vi "Game Controller Teleop.vi"(10 "Match Info":T13={"Autonomous Elapsed Seconds"=0.0, "TeleOp Elapsed Seconds"=0.0, "Disabled Elapsed Seconds"=0.0, "Visited Autonomous"=FALSE, "Visited TeleOp"=FALSE, "Visited Disabled"=FALSE, "Autonomous Settings"={"Autonomous Style"=enum."Independent", "VI Refnum"=refnum}}, 11 "Call Context":T14) -> ()   [LabVIEW 2020]
doc: "This VI is called for each TeleOp packet received from the DS where the robot is not disabled. It is often used to read from the joysticks and update I/O or to update setpoints for timed control loops. It should complete and return within 20 milliseconds or it may miss DS packets."
uses:
  <vilib>/Rock Robotics/WPI/DriverStation/WPI_DriverStationDerivedRobotMode.ctl
  <vilib>/Rock Robotics/WPI/DriverStation/WPI_DriverStationMatch Info.ctl
  Shared Code/TypeDefs/Cluster_Extend HW Outputs.ctl
  Shared Code/TypeDefs/Cluster_FX CloseLoop Values.ctl
  Shared Code/TypeDefs/Cluster_FX Limit Switchs.ctl
  Shared Code/TypeDefs/Cluster_FX Current Values.ctl
  Shared Code/TypeDefs/Cluster_FX Sensor Values.ctl
  Shared Code/TypeDefs/Cluster_FX Integrated Sensor Values.ctl
  Shared Code/TypeDefs/Cluster_Lift_HW Outputs.ctl
  Shared Code/TypeDefs/Cluster_Wrist HW Outputs.ctl
  Shared Code/TypeDefs/Cluster_Pose Positions.ctl
  Systems/MotionMaser/ENUM_Pose List.ctl
  Type Defs/Cluster_Pigeon Tilt Data.ctl
  Shared Code/TypeDefs/ENUM_Tilt State.ctl
  Systems/SwerveDrive/Cluster_CMD_ACT_Data.ctl
  Shared Code/TypeDefs/ENUM_Swerve_CMD_Mode Select.ctl
  Shared Code/TypeDefs/Cluster_CMD_Direction Data.ctl
  Shared Code/TypeDefs/Cluster_Module Velocity-Direction-Rotations.ctl
  Shared Code/TypeDefs/Level_Velocity plus-minus 1.ctl
  Shared Code/TypeDefs/Dial_Compase heading unit circle CCW positive.ctl
  Type Defs/NUM_Rotate Input.ctl
  Shared Code/TypeDefs/Cluster_X-Y.ctl
  Systems/PigeonIMU/Cluster_CMD_SEN_Data.ctl
  Teleop Support/ENUM_Button Select.ctl
  Teleop Support/ENUM_Axes Select.ctl
  Systems/Extention/Cluster_CMD_ACT_Data.ctl
  Shared Code/TypeDefs/ENUM_Extend_CMD_Mode Select.ctl
  Systems/Lift/Cluster_CMD_ACT_Data.ctl
  Shared Code/TypeDefs/ENUM_Lift_CMD_Mode Select.ctl
  Systems/Wrist/Cluster_CMD_ACT_Data.ctl
  Shared Code/TypeDefs/ENUM_Wrist_CMD_Mode Select.ctl
  Systems/Grabber/Cluster_CMD_ACT_Data.ctl
  Shared Code/TypeDefs/ENUM_Grabber_CMD_Mode Select.ctl
  Shared Code/TypeDefs/ENUM_Controller Buzz Select.ctl
  3c76d165-6d6f-4521-944b-83df467126d5.vi
  5b221245-1683-49e4-bbda-b419f5af282c.vi
  8735cd3c-726f-4517-be5d-f0f5cfaf1625.vi
  <vilib>/Rock Robotics/Network Tables/NT Write Boolean.vi
  Systems/Game Controller/Global_SEN_Data Out.vi
  Systems/PigeonIMU/Global_CMD_SEN_Data In.vi
  Systems/Grabber/Global_CMD_ACT_Data In.vi
  Systems/Wrist/Global_CMD_ACT_Data In.vi
  Systems/Extention/Global_ACT_Data Out.vi
  Systems/Lift/Global_ACT_Data Out.vi
  Systems/Wrist/Global_ACT_Data Out.vi
  Systems/Extention/Global_CMD_ACT_Data In.vi
  Systems/Grabber/Global_ACT_Data Out.vi
  Systems/Game Controller/Global_CMD_Data In.vi
  Systems/SwerveDrive/Global_CMD_ACT_Data In.vi
  Systems/Lift/Global_CMD_ACT_Data In.vi
  Systems/PigeonIMU/Global_SEN_Data Out.vi
  Systems/SwerveDrive/Global_ACT_Data Out.vi
  <vilib>/Comparison/Equal/Equal Functor/Equal Functor.lvclass
  Systems/Game Controller/GameController_SEN.lvlib
  Systems/SwerveDrive/SwerveDrive_ACT.lvlib
  Systems/PigeonIMU/PigeonIMU_SEN.lvlib
  Systems/Extention/Extend_ACT.lvlib
  Systems/Lift/Lift_ACT.lvlib
  Systems/Wrist/Wrist_ACT.lvlib
  Systems/Grabber/Grabber_ACT.lvlib
  Systems/MotionMaser/MotionMaster_SubCMD.lvlib
panel:
  out "Rotation Reduction":dbl
  in  "min rotation speed":dbl=0.4
  in  "Balance speed (ft/s)":dbl=10.0
  out "Sen_Pigeon_Tilt Data":T1
  out "Pose":T3
  out "Target  Position Out":T4
  in  "Min Translation Speed (ft/s)":dbl=2.0 format="%#_13g"
  in  "max rotation speed":dbl=0.4
  in  "shoulder speed":dbl=-0.3
  out "ACT_Wrist_HW Output":T5
  out "ACT_Lift_HW Outputs":T11
  out "ACT_Extend_HW Outputs":T12
  out "POSITION":bool
  in  "funny tilt button":bool
  in  "Drive Deadband":dbl=0.25 format="%#_13g"
  in  "Rotation Deadband":dbl=0.15 format="%#_13g"
  in  "Square Throttle?":bool
  in  "Square Joystick Inputs?":bool
  in  "Max Translation Speed (ft/s)":dbl=16.0 format="%#_13g"
  out "POV":i16
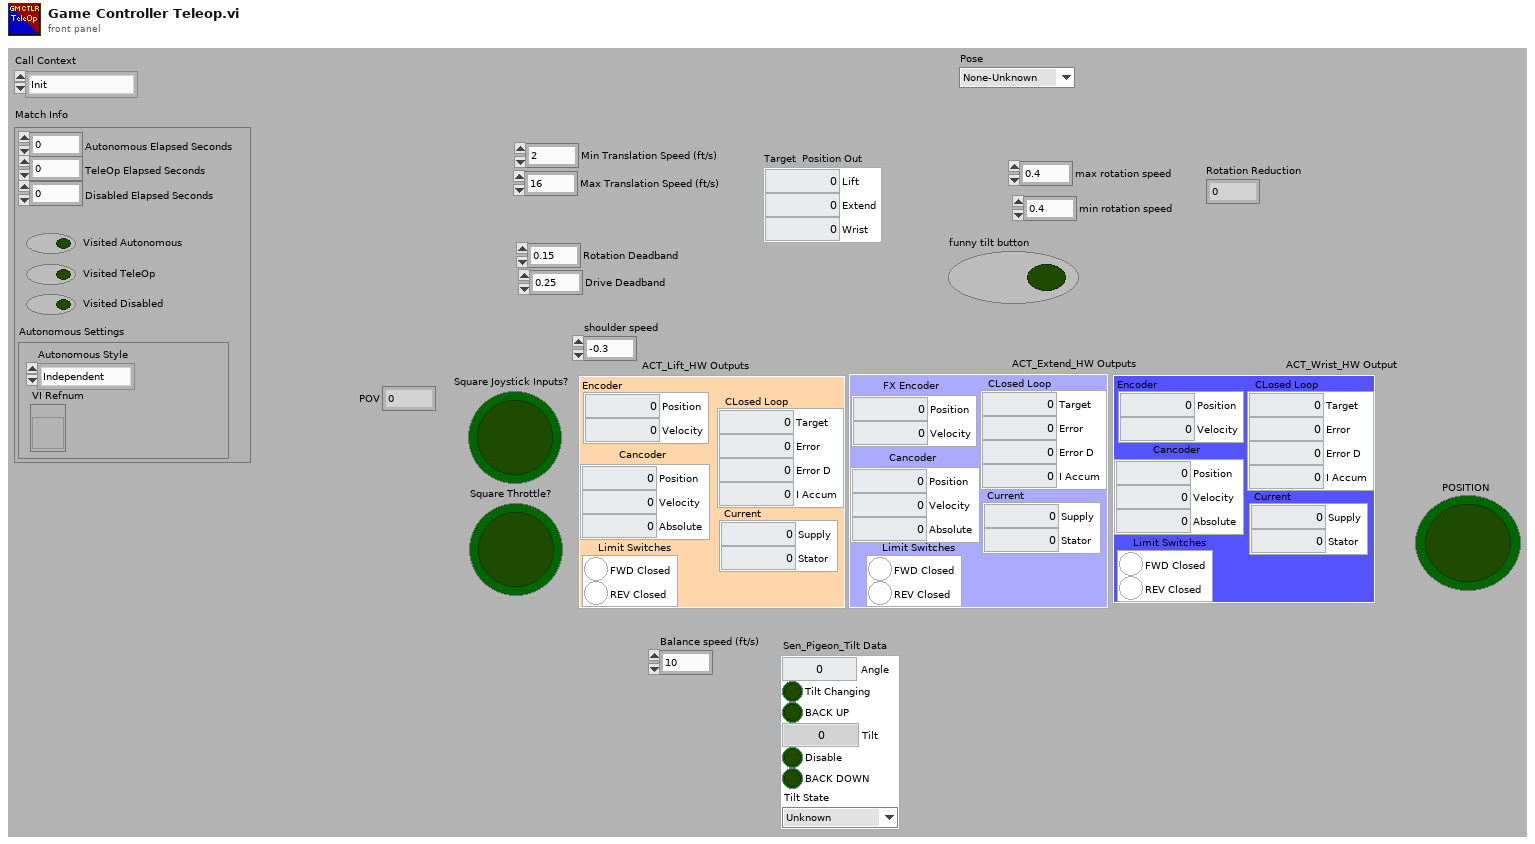
[diagram p1: front panel]
types:
  T1 = typedef "Cluster_Pigeon Tilt Data.ctl" = cluster{"Angle":dbl, "Tilt Changing":bool, "BACK UP":bool, "Tilt":dbl, "Disable":bool, "BACK DOWN":bool, "Tilt State":T2}
  T2 = typedef "ENUM_Tilt State.ctl" = enum16{"Unknown", "Level", "Angle UP from Level", "Level from Angle Up", "Angle Down from Level", "Level from Angle Down"}
  T3 = typedef "MotionMaster_SubCMD.lvlib/ENUM_Pose List.ctl" = enum16{"None-Unknown", "Intake", "Score High", "Score Mid", "Safe Position", "Home Pos"}
  T4 = typedef "Cluster_Pose Positions.ctl" = cluster{"Lift":i32, "Extend":i32, "Wrist":i32}
  T5 = typedef "Cluster_Wrist HW Outputs.ctl" = cluster{"Encoder":T6, "CLosed Loop":T7, "Limit Switches":T8, "Current":T9, "Cancoder":T10}
  T6 = typedef "Cluster_FX Sensor Values.ctl" = cluster{"Position":i32, "Velocity":i32}
  T7 = typedef "Cluster_FX CloseLoop Values.ctl" = cluster{"Target":dbl, "Error":i32, "Error D":dbl, "I Accum":dbl}
  T8 = typedef "Cluster_FX Limit Switchs.ctl" = cluster{"FWD Closed":bool, "REV Closed":bool}
  T9 = typedef "Cluster_FX Current Values.ctl" = cluster{"Supply":dbl, "Stator":dbl}
  T10 = typedef "Cluster_FX Integrated Sensor Values.ctl" = cluster{"Position":dbl, "Velocity":dbl, "Absolute":dbl}
  T11 = typedef "Cluster_Lift_HW Outputs.ctl" = cluster{"Encoder":T6, "CLosed Loop":T7, "Limit Switches":T8, "Current":T9, "Cancoder":T10}
  T12 = typedef "Cluster_Extend HW Outputs.ctl" = cluster{"CLosed Loop":T7, "Limit Switches":T8, "Current":T9, "FX Encoder":T6, "Cancoder":T10}
  T13 = typedef "WPI_DriverStationMatch Info.ctl" = cluster{"Autonomous Elapsed Seconds":dbl, "TeleOp Elapsed Seconds":dbl, "Disabled Elapsed Seconds":dbl, "Visited Autonomous":bool, "Visited TeleOp":bool, "Visited Disabled":bool, "Autonomous Settings":cluster{"Autonomous Style":enum16{"Iterative", "Independent"}, "VI Refnum":refnum<vi>}}
  T14 = typedef "WPI_DriverStationDerivedRobotMode.ctl" = enum16{"Init", "Execute", "Stop"}
  T15 = typedef "ENUM_Button Select.ctl" = enum16{"RightPad Green A", "RightPad Red B", "RightPad Blue X", "RightPad Yellow Y", "Left Bump", "Right Bump", "CenterPad Back", "CenterPad Start", "LeftStick Press", "RightStick Press"}
  T16 = typedef "ENUM_Swerve_CMD_Mode Select.ctl" = enum16{"Coast", "Manual", "Auto Trans Auto Rotate", "Manual Trans Auto Rotate", "Balance", "Stop Brake", "Lock Wheels"}
  T17 = typedef "ENUM_Extend_CMD_Mode Select.ctl" = enum16{"STOP", "Position", "Velocity", "Force Home"}
  T18 = typedef "ENUM_Axes Select.ctl" = enum16{"Left Stick Left (-1) Right (1)", "Left Stick Fwd (-1) Back(1)", "Left Trigger (0-1)", "Right Trigger (0-1)", "Right Stick Left(-1 Right (1)", "Right Stick Fwd(-1) Back (1)"}
  T19 = typedef "NUM_Rotate Input.ctl" = dbl
  T20 = typedef "Dial_Compase heading unit circle CCW positive.ctl" = dbl
  T21 = typedef "ENUM_Grabber_CMD_Mode Select.ctl" = enum16{"STOP", "Intake", "Eject"}
  T22 = typedef "Grabber_ACT.lvlib/Cluster_CMD_ACT_Data.ctl" = cluster{"Mode":T21}
  T23 = typedef "Wrist_ACT.lvlib/Cluster_CMD_ACT_Data.ctl" = cluster{"Mode":T24, "Position (counts)":i32, "Velocity (0-1)":dbl}
  T24 = typedef "ENUM_Wrist_CMD_Mode Select.ctl" = enum16{"STOP", "Position", "Speed"}
  T25 = typedef "Lift_ACT.lvlib/Cluster_CMD_ACT_Data.ctl" = cluster{"Mode":T26, "Position (counts)":i32, "Velocity (0-1)":dbl}
  T26 = typedef "ENUM_Lift_CMD_Mode Select.ctl" = enum16{"STOP", "Position", "Percent out"}
  T27 = typedef "Extend_ACT.lvlib/Cluster_CMD_ACT_Data.ctl" = cluster{"Mode":T17, "Position (counts)":i32, "Velocity (0-1)":dbl}
  T28 = typedef "PigeonIMU_SEN.lvlib/Cluster_CMD_SEN_Data.ctl" = cluster{"Reset":bool, "Disable":bool}
  T29 = typedef "Cluster_Module Velocity-Direction-Rotations.ctl" = cluster{"Velocity":T30, "Angle":T20, "Rotations Count":dbl}
  T30 = typedef "Level_Velocity plus-minus 1.ctl" = dbl
  T31 = typedef "SwerveDrive_ACT.lvlib/Cluster_CMD_ACT_Data.ctl" = cluster{"Mode":T16, "Direction":T32, "Orientation Robot(t) Field(f)":bool, "Max Translation Speed (ft/sec)":dbl, "Rotation Reduction 1-0":dbl, "Rotation Center From Robot Center":T33, "Auto Angle":T20, "Auto Target (ft)":dbl}
  T32 = typedef "Cluster_CMD_Direction Data.ctl" = cluster{"Traverse":T29, "Rotate(Yaw) CCW 1 CW -1":T19}
  T33 = typedef "Cluster_X-Y.ctl" = cluster{"X":dbl, "Y":dbl}
  T34 = typedef "Cluster_Grabber_SW Outputs.ctl" = cluster{"Enabled":bool, "Closed Loop":bool, "Stalled":bool}
  T35 = typedef "GameController_SEN.lvlib/ENUM_SEN_State.ctl" = enum16{"Startup", "Waiting BUZZ ON", "Shutdown", "Buzzing FULL Timed", "Waiting BUZZ OFF", "Buzzing Cycle Count", "Buzzing Intensity"}
  T36 = typedef "ENUM_Controller Buzz Select.ctl" = enum16{"None", "Timed Full ON", "Set Intensity", ".5 Sec Cycle Count"}
  T37 = typedef "Cluster_Config_Balance Data.ctl" = cluster{"BalancePID Ver":u64, "PID":T38}
  T38 = typedef "Cluster_PID Config.ctl" = cluster{"Gains":T39, "Error Allowed":T40, "I Zone":T40, "Max Out":T41, "Max I Accu":T40, "CL Ramp Rate (S)":dbl}
  T39 = typedef "Cluster_PID Gains.ctl" = cluster{"P":dbl, "I":dbl, "D":dbl, "F":dbl}
  T40 = typedef "Cluster_High-Low.ctl" = cluster{"High":dbl, "Low":dbl}
  T41 = typedef "Cluster_FWD  REV Values.ctl" = cluster{"FWD":dbl, "REV":dbl}
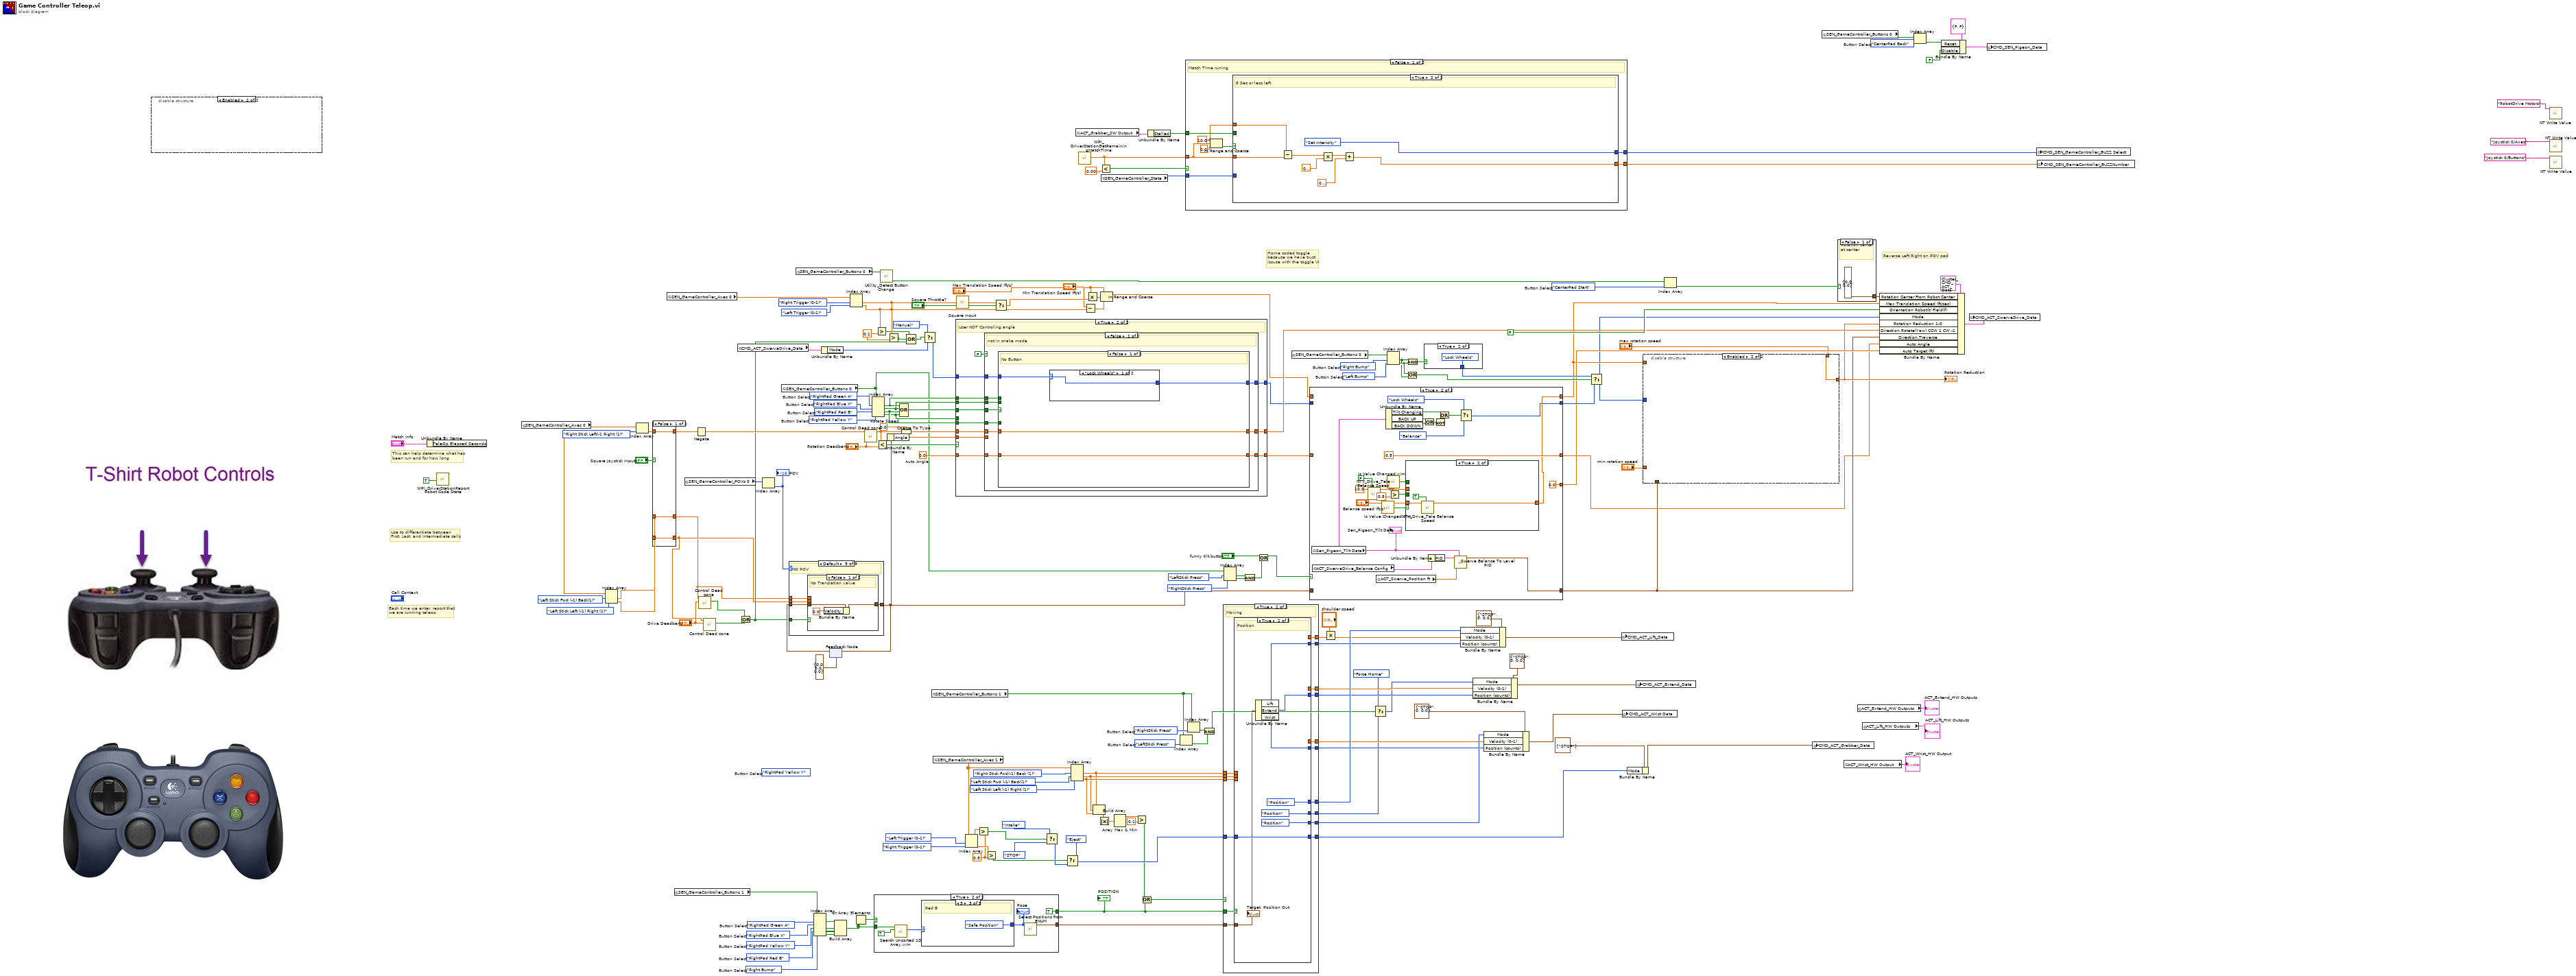
[diagram p0: block diagram]
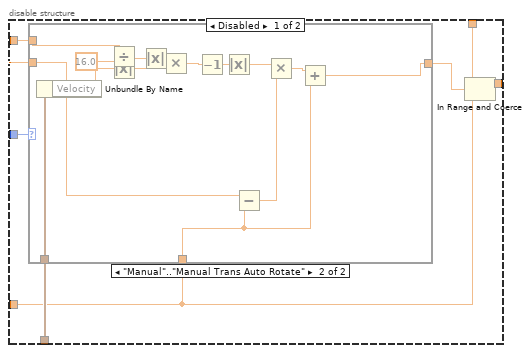
[diagram p2: hidden frame]
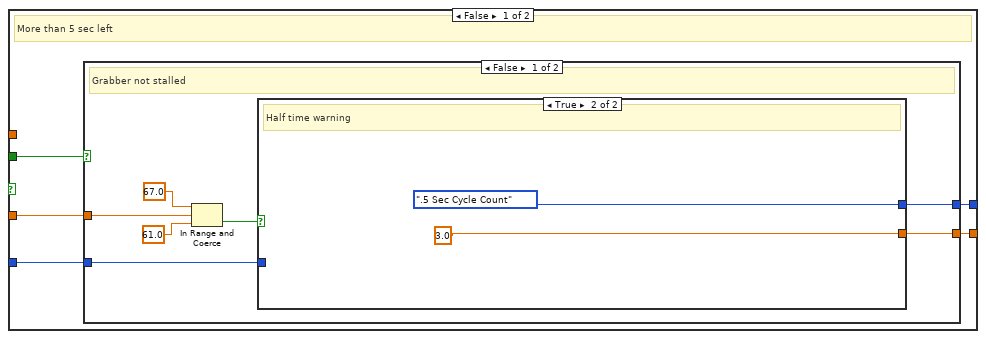
[diagram p4: hidden frame]
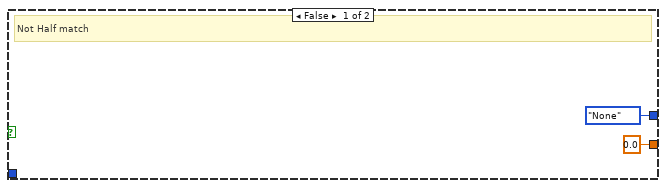
[diagram p5: hidden frame]
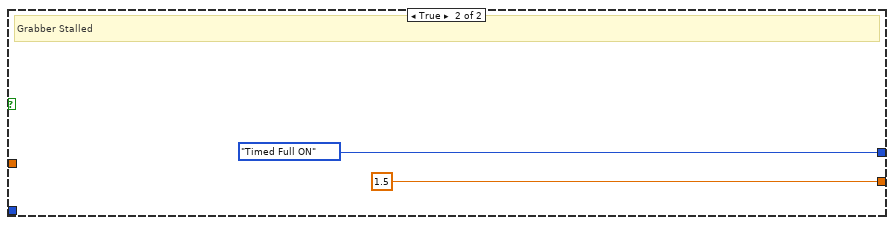
[diagram p6: hidden frame]
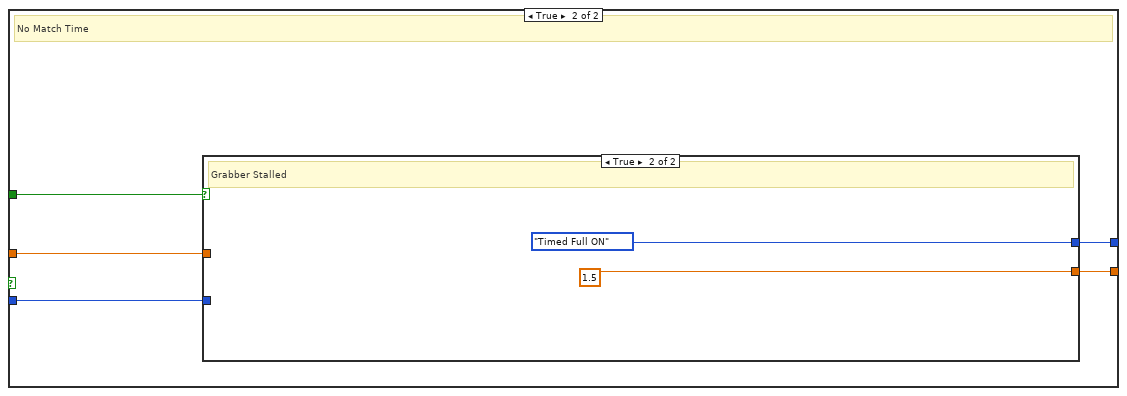
[diagram p7: hidden frame]
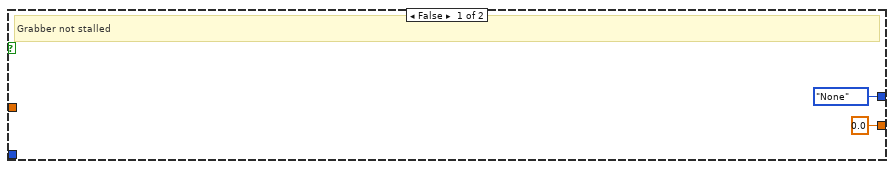
[diagram p8: hidden frame]
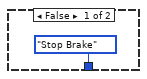
[diagram p9: hidden frame]
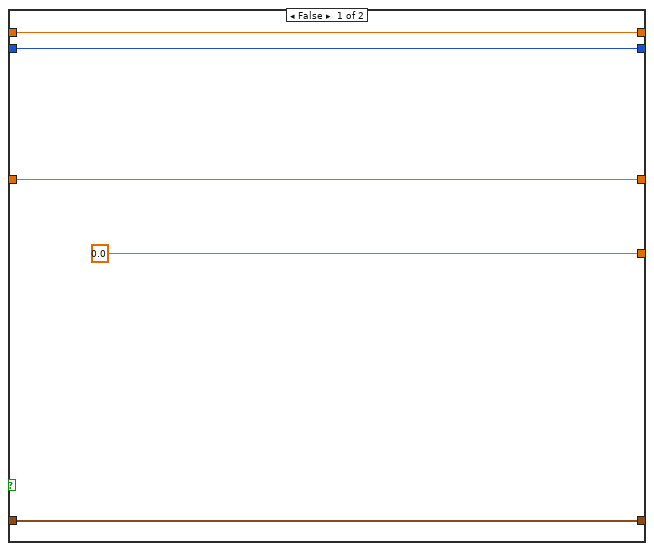
[diagram p10: hidden frame]
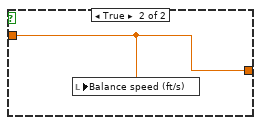
[diagram p13: hidden frame]
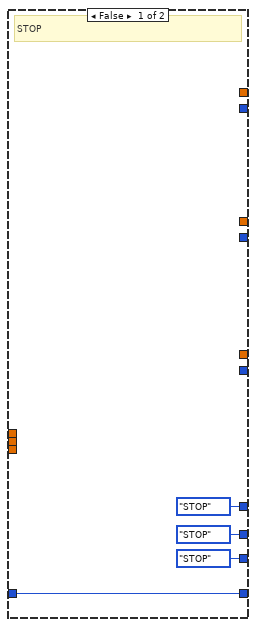
[diagram p14: hidden frame]
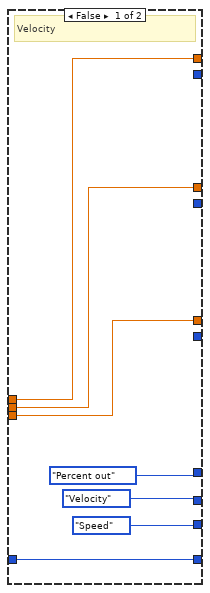
[diagram p15: hidden frame]
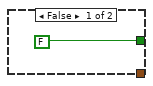
[diagram p16: hidden frame]
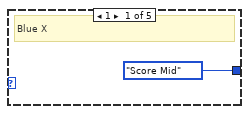
[diagram p17: hidden frame]
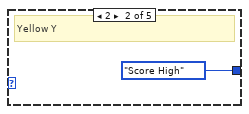
[diagram p18: hidden frame]
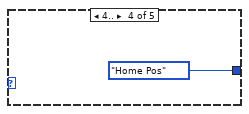
[diagram p19: hidden frame]
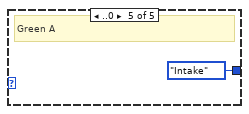
[diagram p20: hidden frame]
diagram:
  w24 = 0.1 ("y")
  w44 = ENUM_Button_Select."Left Bump"  # Button Select
  w53 = ENUM_Button_Select."LeftStick Press"  # Button Select
  w78 = T19 0.0  # Rotate Speed
  w81 = T20 0.0  # Auto Angle
  w84 = ENUM_Button_Select."Right Bump"  # Button Select
  w101 = ENUM_Button_Select."RightPad Red B"  # Button Select
  w102 = ENUM_Button_Select."RightPad Yellow Y"  # Button Select
  w103 = ENUM_Button_Select."RightPad Blue X"  # Button Select
  w104 = ENUM_Button_Select."RightPad Green A"  # Button Select
  (unwired) ENUM_Button_Select."RightPad Yellow Y"  # Button Select
  w111 = 0.9 ("y")
  w147 = ENUM_Button_Select."RightStick Press"  # Button Select
  w157 = ENUM_Button_Select."RightPad Yellow Y"  # Button Select
  w158 = ENUM_Button_Select."RightPad Red B"  # Button Select
  w159 = ENUM_Button_Select."RightPad Blue X"  # Button Select
  w167 = ENUM_Button_Select."CenterPad Start"  # Button Select
  w168 = ENUM_Button_Select."Right Bump"  # Button Select
  w172 = ENUM_Button_Select."CenterPad Back"  # Button Select
  w170 = ENUM_Button_Select."RightPad Green A"  # Button Select
  # "Home coded toggle\nbecause we have trust\nissuse with the toggle VI"
  # "Reverse Left Right on POV pad"
  # "Each time we enter, report that\nwe are running teleop"
  # "Use to differentiate between\nFirst, Last, and Intermediate calls"
  # "This can help determine what has\nbeen run and for how long"
  n1 = disable-structure shown="Enabled" {
    frame Disabled {
      n2 = global read "Global_SEN_Data Out.vi" "SEN_GameController_Axes 1"() -> (w186:dbl[])
      n3 = global read "Global_SEN_Data Out.vi" "SEN_GameController_POVs 1"() -> (w185:i16[])
      n4 = global read "Global_SEN_Data Out.vi" "SEN_GameController_Buttons 1"() -> ()  [unwired: 1 out]
      n5 = Index Array(array=w185) -> ()  [unwired: 1 in, 1 out]
      n6 = Index Array(array=w186) -> ()  [unwired: 1 in, 1 out]
    }
    frame Enabled {
    }
  }
  n7 = Unbundle By Name("Match Info") -> ()  [unwired: 1 out]
  n8 = call <vilib>:"WPI_DriverStationReport Robot Code State.vi"("TeleOp"=TRUE ("Autonomous")) -> ()  [unwired: 10 in, 1 out]
  n9 = global read "Global_SEN_Data Out.vi" "SEN_GameController_Axes 0"() -> (w140:dbl[])
  n10 = Index Array(array=w140, index #1=ENUM_Axes_Select."Left Stick Fwd (-1) Back(1)" ("Axes Select"), index #2=ENUM_Axes_Select."Left Stick Left (-1) Right (1)" ("Axes Select")) -> (element #1=w163:dbl, element #2=w136:dbl)
  n11 = Index Array(array=w140, index=ENUM_Axes_Select."Right Stick Left(-1 Right (1)" ("Axes Select")) -> (element=w138:dbl)
  n12 = case shown="False" "Square Joystick Inputs?" {
    tunnel: [w187 w190] -> w164
    tunnel: [w188 w191] -> w2
    tunnel: [w189 w192] -> w1
    tunnel: w163 -> [w189 w195]
    tunnel: w138 -> [w187 w193]
    tunnel: w136 -> [w188 w194]
    frame False {
    }
    frame True {
      n13 = call "Square Input.vi"("Input"=w193) -> ("Output Squared"=w190:dbl)
      n14 = call "Square Input.vi"("Input"=w195) -> ("Output Squared"=w192:dbl)
      n15 = call "Square Input.vi"("Input"=w194) -> ("Output Squared"=w191:dbl)
    }
  }
  n16 = global read "Global_SEN_Data Out.vi" "SEN_GameController_Axes 0"() -> (w143:dbl[])
  n17 = global read "Global_SEN_Data Out.vi" "SEN_GameController_Buttons 1"() -> (w86:bool[])
  n18 = global read "Global_SEN_Data Out.vi" "SEN_GameController_POVs 0"() -> (w179:i16[])
  n19 = Negate(x=w164) -> (-x=w75:dbl)
  n20 = call "Control Dead zone.vi"("dead zone"="Drive Deadband", "control Value"=w1) -> ("Active"=w71:bool)  [unwired: 8 in, 1 out]
  n21 = call "Control Dead zone.vi"("dead zone"="Drive Deadband", "control Value"=w2) -> ("Active"=w72:bool)  [unwired: 8 in, 1 out]
  n22 = global read "Global_CMD_ACT_Data In.vi" "CMD_ACT_SwerveDrive_Data"() -> (w29:T31)
  n23 = Or(x=w71, y=w72) -> (x .or. y?=w19:bool)
  n24 = Index Array(array=w179) -> (element=w146:i16)  [unwired: 1 in]
  "POV" <- w146
  n25 = global read "Global_SEN_Data Out.vi" "SEN_GameController_Buttons 0"() -> (w18:bool[])
  n26 = global read "Global_SEN_Data Out.vi" "SEN_GameController_Buttons 0"() -> (w55:bool[])
  n27 = Index Array(array=w86, index #1=w104, index #2=w103, index #3=w102, index #4=w101, index #5=w84) -> (element #1=w100:bool, element #2=w99:bool, element #3=w98:bool, element #4=w97:bool, element #5=w83:bool)
  n28 = Unbundle By Name(w29) -> ("Mode"=w22:T16)
  n29 = feedback #1(T29 {"Velocity"=0.0, "Angle"=0.0, "Rotations Count"=0.0} ("Polar Out")) -> (w74:T29)
  n30 = case shown="Default" w146 {
    tunnel: w1 -> [_ _ _ _ _ _ _ _ w232]
    tunnel: w2 -> [_ _ _ _ _ _ _ _ w231]
    tunnel: w74 -> [w199 w203 w207 w211 w215 w219 w223 w227 w230]
    tunnel: [w196 w200 w204 w208 w212 w216 w220 w224 w229] -> w11
    tunnel: w19 -> [_ _ _ _ _ _ _ _ w228]
    frame 0 {
      # "POV Forward"
      n31 = Bundle By Name(cluster=w199, "Velocity"=T30 1.0, "Angle"=T20 0.0) -> (w196:T29)
    }
    frame 45 {
      # "POV Forward Right"
      n32 = Bundle By Name(cluster=w203, "Velocity"=T30 1.0, "Angle"=T20 0.875) -> (w200:T29)
    }
    frame 90 {
      # "POV Right"
      n33 = Bundle By Name(cluster=w207, "Velocity"=T30 1.0, "Angle"=T20 0.75) -> (w204:T29)
    }
    frame 135 {
      # "POV Back Right"
      n34 = Bundle By Name(cluster=w211, "Velocity"=T30 1.0, "Angle"=T20 0.625) -> (w208:T29)
    }
    frame 180 {
      # "POV Back"
      n35 = Bundle By Name(cluster=w215, "Velocity"=T30 1.0, "Angle"=T20 0.5) -> (w212:T29)
    }
    frame 225 {
      # "POV Back Left"
      n36 = Bundle By Name(cluster=w219, "Velocity"=T30 1.0, "Angle"=T20 0.375) -> (w216:T29)
    }
    frame 270 {
      # "POV Left"
      n37 = Bundle By Name(cluster=w223, "Velocity"=T30 1.0, "Angle"=T20 0.25) -> (w220:T29)
    }
    frame 315 {
      # "POV Forward Left"
      n38 = Bundle By Name(cluster=w227, "Velocity"=T30 1.0, "Angle"=T20 0.125) -> (w224:T29)
    }
    frame Default {
      # "NO POV"
      n39 = case shown="False" w228 {
        tunnel: w232 -> [_ w242]
        tunnel: w231 -> [_ w241]
        tunnel: w230 -> [w234 _]
        tunnel: [w235 w238] -> w229
        frame False {
          # "No Translation value"
          n40 = Bundle By Name(cluster=w234, "Velocity"=T30 0.0) -> (w235:T29)
        }
        frame True {
          # "Tranlation Value above threshold"
          n41 = Negate(x=w241) -> (-x=w237:dbl)
          n42 = Negate(x=w242) -> (-x=w236:dbl)
          n43 = Bundle By Name(cluster=T33 {"X"=0.0, "Y"=0.0} ("XY Velocities"), "X"=w236, "Y"=w237) -> (w240:T33)
          n44 = call "Convert XY To Polar Velocities.vi"("XY Velocities"=w240) -> ("Polar Out"=w238:T29)  [unwired: 10 in]
        }
      }
    }
  }
  n45 = feedback-in #1(w11) -> ()
  n46 = Build Array(w100, w99, w98, w97, w83) -> (w95:bool[])
  n47 = Index Array(array=w143, index #1=ENUM_Axes_Select."Right Trigger (0-1)" ("Axes Select"), index #2=ENUM_Axes_Select."Left Trigger (0-1)" ("Axes Select")) -> (element #1=w27:dbl, element #2=w28:dbl)
  n48 = Or Array Elements(Boolean array=w95) -> (logical OR=w96:bool)
  n49 = call "Control Dead zone.vi"("dead zone"="Rotation Deadband", "control Value"=w75) -> ("output Value"=w80:dbl)  [unwired: 8 in, 1 out]
  n50 = Index Array(array=w18, index #1=w170, index #2=w159, index #3=w158, index #4=w157) -> (element #1=w155:bool, element #2=w152:bool, element #3=w154:bool, element #4=w153:bool)
  n51 = case shown="True" w96 {
    tunnel: [_ w245] -> w105
    tunnel: w95 -> [_ w249]
    tunnel: [FALSE TRUE] -> w61
    frame False {
    }
    frame True {
      n52 = call "Search Unsorted 1D Array.vim"("element"=TRUE, "unsorted 1D array"=w249) -> ("index of element"=w247:i32)  [unwired: 9 in]
      n53 = case shown="3" w247 {
        tunnel: [ENUM_Pose_List."Score Mid" ("Pose") ENUM_Pose_List."Score High" ("Pose") ENUM_Pose_List."Safe Position" ("Pose") ENUM_Pose_List."Home Pos" ("Pose") ENUM_Pose_List."Intake" ("Pose")] -> w244
        frame 1 {
          # "Blue X"
        }
        frame 2 {
          # "Yellow Y"
        }
        frame 3 {
          # "Red B"
        }
        frame 4.. {
        }
        frame ..0 {
          # "Green A"
        }
      }
      "Pose" <- w244
      n54 = call "Select Positions from ENUM.vi"("Pose"=w244) -> ("Selectet  Position Out"=w245:T4)  [unwired: 10 in]
    }
  }
  "POSITION" <- w61
  n55 = Greater?(x=w28, y=w24) -> (0:w25:bool)
  n56 = Less?(x=w80, y="Rotation Deadband") -> (x < y?=w150:bool)
  n57 = call "Utility_Detect Button Change.vi"("HW_Joystick_Buttons"=w55) -> ("Toggle On Rising Out"=w54:bool[])  [unwired: 6 in, 4 out]
  n58 = Greater?(x=w27, y=w24) -> (0:w26:bool)
  n59 = Unbundle By Name(w11) -> ("Angle"=w145:T20)
  n60 = Compound Arithmetic op=OR(w155, w152, w154, w153) -> (w156:bool)
  n61 = Coerce To Type(0:w80, 1:w78) -> (2:w79:T19)
  n62 = Compound Arithmetic op=OR(w25, w26, w19) -> (w23:bool)
  n63 = Select(t=ENUM_Swerve_CMD_Mode_Select."Manual", s=w23, f=w22) -> (s? t:f=w21:T16)
  n64 = global read "Global_SEN_Data Out.vi" "SEN_GameController_Buttons 1"() -> (w52:bool[])
  n65 = global read "Global_SEN_Data Out.vi" "SEN_GameController_Axes 1"() -> (w116:dbl[])
  n66 = case shown="True" w150 {
    tunnel: w79 -> [w255 w269]
    tunnel: w156 -> [_ w268]
    tunnel: w155 -> [_ w267]
    tunnel: w154 -> [_ w266]
    tunnel: w153 -> [_ _]
    tunnel: w152 -> [_ w265]
    tunnel: [w255 w264] -> w82
    tunnel: w145 -> [_ w263]
    tunnel: [ENUM_Swerve_CMD_Mode_Select."Manual" ("Mode") w260] -> w77
    tunnel: w81 -> [w256 w262]
    tunnel: [w256 w261] -> w76
    tunnel: w21 -> [_ w258]
    frame False {
      # "User Controling Angle"
    }
    frame True {
      # "User NOT Controling angle"
      n67 = case shown="False" FALSE {
        tunnel: w269 -> [w271 w303]
        tunnel: w268 -> [w277 w302]
        tunnel: w267 -> [w276 w301]
        tunnel: w266 -> [w275 w300]
        tunnel: w265 -> [w274 w299]
        tunnel: [w271 w298] -> w264
        tunnel: w263 -> [w273 _]
        tunnel: w262 -> [_ w297]
        tunnel: [w272 w296] -> w261
        tunnel: [ENUM_Swerve_CMD_Mode_Select."Manual Trans Auto Rotate" ("Mode") w295] -> w260
        tunnel: w258 -> [_ w294]
        frame True {
          # "in snake mode"
          n68 = case shown="True" w277 {
            tunnel: w276 -> [_ w284]
            tunnel: w275 -> [_ w283]
            tunnel: w274 -> [_ w282]
            tunnel: [w278 w280] -> w272
            tunnel: w273 -> [w278 w279]
            frame False {
              # "No Button"
            }
            frame True {
              # "a,b,x,y Button Pressed"
              n69 = case shown="True" w284 {
                tunnel: w283 -> [w287 _]
                tunnel: [w286 w293] -> w281
                tunnel: w282 -> [w285 _]
                frame False {
                  n70 = case shown="True" w285 {
                    tunnel: w287 -> [w289 _]
                    tunnel: [w288 w292] -> w286
                    frame False {
                      n71 = case shown="False" w289 {
                        tunnel: [w290 w291] -> w288
                        frame False {
                          w290 = T20 0.0  # Auto Angle
                          # "Y"
                        }
                        frame True {
                          w291 = T20 0.25  # Auto Angle
                          # "B"
                        }
                      }
                    }
                    frame True {
                      w292 = T20 0.75  # Auto Angle
                      # "X"
                    }
                  }
                }
                frame True {
                  w293 = T20 0.5  # Auto Angle
                  # "A"
                }
              }
              n72 = Subtract(x=w279, y=w281) -> (x-y=w280:T20)
            }
          }
        }
        frame False {
          # "not in snake mode"
          n73 = case shown="False" w302 {
            tunnel: w303 -> [w307 w311]
            tunnel: w301 -> [_ w316]
            tunnel: w300 -> [_ w315]
            tunnel: w299 -> [_ w314]
            tunnel: [w307 w311] -> w298
            tunnel: w297 -> [w306 w312]
            tunnel: [w306 w313] -> w296
            tunnel: [w305 ENUM_Swerve_CMD_Mode_Select."Manual Trans Auto Rotate" ("Mode")] -> w295
            tunnel: w294 -> [w304 _]
            frame False {
              # "No Button"
              n74 = case shown="\"Lock Wheels\"" w304 {
                selector: w304 -> [w308 _]
                tunnel: [w308 ENUM_Swerve_CMD_Mode_Select."Manual" ("Mode")] -> w305
                frame "Lock Wheels" {
                }
                frame Default {
                }
              }
            }
            frame True {
              # "a,b,x,y Button Pressed"
              n75 = case shown="True" w316 {
                tunnel: w315 -> [w320 _]
                tunnel: [w319 w327] -> w313
                tunnel: w314 -> [w318 _]
                tunnel: w312 -> [w317 _]
                frame False {
                  n76 = case shown="True" w318 {
                    tunnel: w320 -> [w323 _]
                    tunnel: [w322 w326] -> w319
                    tunnel: w317 -> [w321 _]
                    frame False {
                      n77 = case shown="True" w323 {
                        tunnel: [w324 w325] -> w322
                        tunnel: w321 -> [w324 _]
                        frame False {
                          # "Y"
                        }
                        frame True {
                          w325 = T20 0.75  # Auto Angle
                          # "B"
                        }
                      }
                    }
                    frame True {
                      w326 = T20 0.25  # Auto Angle
                      # "X"
                    }
                  }
                }
                frame True {
                  w327 = T20 0.5  # Auto Angle
                  # "A"
                }
              }
            }
          }
        }
      }
    }
  }
  n78 = call "Square Input.vi"("Input"=w27) -> ("Output Squared"=w151:dbl)
  n79 = Index Array(array=w116, index #1=ENUM_Axes_Select."Left Trigger (0-1)" ("Axes Select"), index #2=ENUM_Axes_Select."Right Trigger (0-1)" ("Axes Select")) -> (element #1=w113:dbl, element #2=w112:dbl)
  n80 = Greater?(x=w113, y=w111) -> (0:w110:bool)
  n81 = Greater?(x=w112, y=w111) -> (0:w109:bool)
  n82 = Select(t=w151, s="Square Throttle?", f=w27) -> (s? t:f=w160:dbl)
  n83 = Select(t=ENUM_Grabber_CMD_Mode_Select."Intake" ("Mode"), s=w110, f=ENUM_Grabber_CMD_Mode_Select."STOP" ("Mode")) -> (s? t:f=w117:T21)
  n84 = Select(t=ENUM_Grabber_CMD_Mode_Select."Eject" ("Mode"), s=w109, f=w117) -> (s? t:f=w94:T21)
  n85 = Index Array(array=w116, index #1=ENUM_Axes_Select."Right Stick Fwd(-1) Back (1)" ("Axes Select"), index #2=ENUM_Axes_Select."Left Stick Fwd (-1) Back(1)" ("Axes Select"), index #3=ENUM_Axes_Select."Left Stick Left (-1) Right (1)" ("Axes Select")) -> (element #1=w68:dbl, element #2=w69:dbl, element #3=w70:dbl)
  n86 = global read "Global_ACT_Data Out.vi" "ACT_Grabber_SW Output"() -> (w31:T34)
  n87 = call <vilib>:"WPI_DriverStationGetRemainingMatchTime.vi"() -> ("Match Time(s)"=w33:sgl)  [unwired: 10 in, 1 out]
  n88 = Subtract(x="Min Translation Speed (ft/s)", y=w28) -> (x-y=w57:dbl)
  n89 = Multiply(x="Max Translation Speed (ft/s)", y=w160) -> (x*y=w60:dbl)
  n90 = Build Array(w68, w69, w70) -> (w67:dbl[])
  n91 = Absolute Value(x=w67) -> (abs(x)=w66:dbl[])
  n92 = Less?(x=w33, y=sgl 0.01 ("x")) -> (x < y?=w35:bool)
  n93 = In Range and Coerce(upper limit="Max Translation Speed (ft/s)", x=w60, lower limit=w57) -> (coerced(x)=w59:dbl)  [unwired: 1 out]
  n94 = global read "Global_SEN_Data Out.vi" "SEN_GameController_State"() -> (w34:T35)
  n95 = Array Max & Min(array=w66) -> (max value=w65:dbl)  [unwired: 3 out]
  n96 = Greater?(x=w65, y=0.1) -> (0:w63:bool)
  n97 = Or(x=w63, y=w61) -> (x .or. y?=w62:bool)
  n98 = Unbundle By Name(w31) -> ("Stalled"=w30:bool)
  n99 = Index Array(array=w52, index=w53) -> (element=w50:bool)
  n100 = case shown="False" w35 {
    tunnel: [w333 w366] -> w37
    tunnel: [w332 w363] -> w36
    tunnel: w30 -> [w331 w365]
    tunnel: w33 -> [w330 w364]
    tunnel: w34 -> [w328 w362]
    frame False {
      w329 = sgl 10.0 ("upper limit")
      # "Match Time runing"
      n101 = In Range and Coerce(upper limit=w329, x=w330, lower limit=sgl 0.0) -> (In Range?=w334:bool)  [unwired: 1 out]
      n102 = case shown="True" w334 {
        tunnel: w330 -> [w338 w360]
        tunnel: [w339 ENUM_Controller_Buzz_Select."Set Intensity" ("CMD_SEN_GameController_BUZZ Select")] -> w333
        tunnel: [w337 w354] -> w332
        tunnel: w331 -> [w340 _]
        tunnel: w329 -> [_ w358]
        tunnel: w328 -> [w336 _]
        frame False {
          # "More than 5 sec left"
          n103 = case shown="False" w340 {
            tunnel: [w343 ENUM_Controller_Buzz_Select."Timed Full ON" ("CMD_SEN_GameController_BUZZ Select")] -> w339
            tunnel: w338 -> [w345 _]
            tunnel: [w342 sgl 1.5] -> w337
            tunnel: w336 -> [w341 _]
            frame False {
              # "Grabber not stalled"
              n104 = In Range and Coerce(upper limit=sgl 67.0, x=w345, lower limit=sgl 61.0) -> (In Range?=w344:bool)  [unwired: 1 out]
              n105 = case shown="True" w344 {
                tunnel: [ENUM_Controller_Buzz_Select."None" ("CMD_SEN_GameController_BUZZ Select") ENUM_Controller_Buzz_Select.".5 Sec Cycle Count" ("CMD_SEN_GameController_BUZZ Select")] -> w343
                tunnel: [sgl 0.0 sgl 3.0] -> w342
                tunnel: w341 -> [_ _]
                frame False {
                  # "Not Half match"
                }
                frame True {
                  # "Half time warning"
                }
              }
            }
            frame True {
              # "Grabber Stalled"
            }
          }
        }
        frame True {
          # "5 Sec or less left"
          n106 = Subtract(x=w358, y=w360) -> (x-y=w359:sgl)
          n107 = Multiply(x=w359, y=sgl 0.6) -> (x*y=w357:sgl)
          n108 = Add(x=w357, y=sgl 0.4) -> (x+y=w354:sgl)
        }
      }
    }
    frame True {
      # "No Match Time"
      n109 = case shown="True" w365 {
        tunnel: [ENUM_Controller_Buzz_Select."None" ("CMD_SEN_GameController_BUZZ Select") ENUM_Controller_Buzz_Select."Timed Full ON" ("CMD_SEN_GameController_BUZZ Select")] -> w366
        tunnel: w364 -> [_ _]
        tunnel: [sgl 0.0 sgl 1.5] -> w363
        tunnel: w362 -> [_ _]
        frame False {
          # "Grabber not stalled"
        }
        frame True {
          # "Grabber Stalled"
        }
      }
    }
  }
  n110 = Index Array(array=w52, index=w147) -> (element=w51:bool)
  n111 = And(x=w51, y=w50) -> (x .and. y?=w49:bool)
  n112 = case shown="True" w62 {
    tunnel: [ENUM_Wrist_CMD_Mode_Select."STOP" ("Mode") w390] -> w125
    tunnel: [ENUM_Extend_CMD_Mode_Select."STOP" ("Mode") w389] -> w47
    tunnel: [ENUM_Lift_CMD_Mode_Select."STOP" ("Mode") w388] -> w124
    tunnel: [w371 w387] -> w121
    tunnel: [_ w385] -> w108
    tunnel: w68 -> [_ w384]
    tunnel: [_ w383] -> w107
    tunnel: w69 -> [_ w382]
    tunnel: w70 -> [_ w381]
    tunnel: [_ w380] -> w106
    tunnel: w105 -> [_ w379]
    tunnel: w94 -> [w371 w386]
    tunnel: [_ w378] -> w90
    tunnel: [_ w377] -> w89
    tunnel: [_ w376] -> w88
    tunnel: w61 -> [_ w375]
    frame False {
      # "STOP"
    }
    frame True {
      # "Moving"
      n113 = case shown="True" w375 {
        tunnel: [ENUM_Wrist_CMD_Mode_Select."Speed" ("Mode") ENUM_Wrist_CMD_Mode_Select."Position" ("Mode")] -> w390
        tunnel: [ENUM_Extend_CMD_Mode_Select."Velocity" ("Mode") ENUM_Extend_CMD_Mode_Select."Position" ("Mode")] -> w389
        tunnel: [ENUM_Lift_CMD_Mode_Select."Percent out" ("Mode") ENUM_Lift_CMD_Mode_Select."Position" ("Mode")] -> w388
        tunnel: [w394 w402] -> w387
        tunnel: w386 -> [w394 w402]
        tunnel: [w393 _] -> w385
        tunnel: w384 -> [w393 _]
        tunnel: [w392 _] -> w383
        tunnel: w382 -> [w392 _]
        tunnel: w381 -> [w391 _]
        tunnel: [w391 _] -> w380
        tunnel: w379 -> [_ w401]
        tunnel: [_ w400] -> w378
        tunnel: [_ w399] -> w377
        tunnel: [_ w398] -> w376
        frame False {
          # "Velocity"
        }
        frame True {
          # "Position"
          n114 = Unbundle By Name(w401) -> ("Lift"=w399:i32, "Extend"=w400:i32, "Wrist"=w398:i32)
          "Target  Position Out" <- w401
        }
      }
    }
  }
  n115 = Index Array(array=w18, index #1=ENUM_Button_Select."LeftStick Press" ("Button Select"), index #2=ENUM_Button_Select."RightStick Press" ("Button Select")) -> (element #1=w14:bool, element #2=w15:bool)
  n116 = And(x=w14, y=w15) -> (x .and. y?=w13:bool)
  n117 = Or(x="funny tilt button", y=w13) -> (x .or. y?=w12:bool)
  n118 = global read "Global_SEN_Data Out.vi" "SEN_GameController_Buttons 0"() -> (w169:bool[])
  n119 = case shown="True" w12 {
    tunnel: w11 -> [w410 _]
    tunnel: [w410 w435] -> w8
    tunnel: w77 -> [w409 _]
    tunnel: [w409 w422] -> w43
    tunnel: w76 -> [w408 _]
    tunnel: [w408 T20 0.5 ("Auto Angle")] -> w3
    tunnel: w59 -> [w407 _]
    tunnel: [w407 w416] -> w7
    tunnel: [0.0 ("Auto Target (ft)") 0.0 ("Auto Target (ft)")] -> w10
    frame False {
    }
    frame True {
      n120 = global read "Global_SEN_Data Out.vi" "Sen_Pigeon_Tilt Data"() -> (w428:T1)
      "Sen_Pigeon_Tilt Data" <- w428
      n121 = global read "Global_ACT_Data Out.vi" "ACT_SwerveDrive_Balance Config"() -> (w434:T37)
      n122 = call "NTV_Drive_Tele Balance Speed.vi"("Read(f) Write(t)"=FALSE, "Balance Speed"=10.0) -> ("Balance Speed"=w412:dbl)  [unwired: 9 in]
      n123 = global read "Global_ACT_Data Out.vi" "ACT_Swerve_Position ft"() -> (w432:dbl)
      n124 = call "Is Value Changed.vim"("value"="Balance speed (ft/s)") -> ("changed or first call?"=w413:bool)
      n125 = Unbundle By Name(w428) -> ("Tilt Changing"=w426:bool, "BACK UP"=w431:bool, "BACK DOWN"=w429:bool)
      n126 = call "Is Value Changed.vim"("value"=w412) -> ("changed or first call?"=w411:bool)
      n127 = Greater?(x=w412, y=0.5) -> (0:w415:bool)
      n128 = case shown="True" w413 {
        tunnel: "Balance speed (ft/s)" -> [w438 w449]
        tunnel: [w437 w447] -> w416
        tunnel: w415 -> [w440 _]
        tunnel: w412 -> [w439 _]
        tunnel: w411 -> [w436 _]
        frame False {
          n129 = case shown="True" w440 {
            tunnel: w439 -> [_ w443]
            tunnel: [w441 w442] -> w437
            tunnel: w438 -> [w441 _]
            tunnel: w436 -> [_ w444]
            frame False {
            }
            frame True {
              n130 = case shown="False" w444 {
                tunnel: w443 -> [w445 w446]
                tunnel: [w445 w446] -> w442
                frame False {
                }
                frame True {
                  n131 = local write "Balance speed (ft/s)"(w446) -> ()
                }
              }
            }
          }
        }
        frame True {
          n132 = call "NTV_Drive_Tele Balance Speed.vi"("Read(f) Write(t)"=TRUE, "Balance Speed"=w449) -> ("Balance Speed"=w447:dbl)  [unwired: 9 in]
        }
      }
      n133 = Or(x=w431, y=w429) -> (x .or. y?=w430:bool)
      n134 = Unbundle By Name(w434) -> ("PID"=w433:T38)
      n135 = Not(x=w430) -> (.not. x?=w427:bool)
      n136 = Or(x=w426, y=w427) -> (x .or. y?=w425:bool)
      n137 = call "Swerve Balance To Level PID.vi"("Yaw Data"=w428, "Position ft"=w432, "Tilt PID Config"=w433) -> ("Output Cluster Out"=w435:T29)  [unwired: 6 in, 2 out]
      n138 = Select(t=ENUM_Swerve_CMD_Mode_Select."Lock Wheels" ("Mode"), s=w425, f=ENUM_Swerve_CMD_Mode_Select."Balance" ("Mode")) -> (s? t:f=w422:T16)
    }
  }
  n139 = Multiply(x="shoulder speed", y=w108) -> (x*y=w87:dbl)
  n140 = Select(t=ENUM_Extend_CMD_Mode_Select."Force Home" ("Mode"), s=w49, f=w47) -> (s? t:f=w46:T17)
  n141 = Index Array(array=w169, index #1=w168, index #2=w44) -> (element #1=w40:bool, element #2=w41:bool)
  n142 = Or(x=w41, y=w40) -> (x .or. y?=w39:bool)
  n143 = And(x=w40, y=w41) -> (x .and. y?=w38:bool)
  n144 = case shown="True" w38 {
    tunnel: [ENUM_Swerve_CMD_Mode_Select."Stop Brake" ("t") ENUM_Swerve_CMD_Mode_Select."Lock Wheels" ("t")] -> w42
    frame False {
    }
    frame True {
    }
  }
  n145 = Bundle By Name(cluster=T25 {"Mode"=enum."STOP", "Position (counts)"=0, "Velocity (0-1)"=0.0} ("CMD_ACT_Template_Data"), "Mode"=w124, "Velocity (0-1)"=w87, "Position (counts)"=w89) -> (w131:T25)
  n146 = Bundle By Name(cluster=T27 {"Mode"=enum."STOP", "Position (counts)"=0, "Velocity (0-1)"=0.0} ("CMD_ACT_Template_Data"), "Mode"=w46, "Velocity (0-1)"=w107, "Position (counts)"=w90) -> (w133:T27)
  n147 = Bundle By Name(cluster=T23 {"Mode"=enum."STOP", "Position (counts)"=0, "Velocity (0-1)"=0.0} ("CMD_ACT_Template_Data"), "Mode"=w125, "Velocity (0-1)"=w106, "Position (counts)"=w88) -> (w129:T23)
  n148 = Select(t=w42, s=w39, f=w43) -> (s? t:f=w6:T16)
  n149 = global write "Global_CMD_ACT_Data In.vi" "CMD_ACT_Lift_Data"(w131) -> ()
  n150 = global write "Global_CMD_ACT_Data In.vi" "CMD_ACT_Wrist Data"(w129) -> ()
  n151 = Bundle By Name(cluster=T22 {"Mode"=enum."STOP"} ("CMD_Wrist_Template_Data"), "Mode"=w121) -> (w122:T22)
  n152 = global write "Global_CMD_ACT_Data In.vi" "CMD_ACT_Extend_Data"(w133) -> ()
  n153 = disable-structure shown="Enabled" {
    disable-tunnel: [w458 w475] -> w9
    disable-tunnel: w8 -> [w457 _]
    disable-tunnel: w7 -> [w456 _]
    disable-tunnel: w6 -> [w455 _]
    disable-tunnel: "max rotation speed" -> [w453 w475]
    disable-tunnel: "min rotation speed" -> [w452 _]
    frame Disabled {
      n154 = case shown="\"Manual\"..\"Manual Trans Auto Rotate\"" w455 {
        tunnel: w457 -> [_ w474]
        tunnel: w456 -> [_ w473]
        tunnel: [w459 w465] -> w454
        tunnel: w453 -> [w459 w468]
        tunnel: w452 -> [_ w463]
        frame "Coast", "Balance".."Lock Wheels" {
        }
        frame "Manual".."Manual Trans Auto Rotate" {
          n155 = Unbundle By Name(w474) -> ("Velocity"=w470:T30)
          n156 = Divide(x=w473, y=16.0) -> (x/y=w471:dbl)
          n157 = Absolute Value(x=w470) -> (abs(x)=w461:T30)
          n158 = Absolute Value(x=w471) -> (abs(x)=w462:dbl)
          n159 = Multiply(x=w462, y=w461) -> (x*y=w469:T30)
          n160 = Decrement(x=w469) -> (x-1=w467:T30)
          n161 = Absolute Value(x=w467) -> (abs(x)=w460:T30)
          n162 = Subtract(x=w468, y=w463) -> (x-y=w466:dbl)
          n163 = Multiply(x=w460, y=w466) -> (x*y=w464:T30)
          n164 = Add(x=w464, y=w463) -> (x+y=w465:T30)
        }
      }
      n165 = In Range and Coerce(upper limit=w453, x=w454, lower limit=w452) -> (coerced(x)=w458:T30)  [unwired: 1 out]
    }
    frame Enabled {
    }
  }
  "Rotation Reduction" <- w9
  n166 = Index Array(array=w54, index=w167) -> (element=w166:bool)
  n167 = global write "Global_CMD_ACT_Data In.vi" "CMD_ACT_Grabber_Data"(w122) -> ()
  n168 = global read "Global_SEN_Data Out.vi" "SEN_GameController_Buttons 0"() -> (w142:bool[])
  n169 = case shown="False" w166 {
    tunnel: [T33 {"X"=0.0, "Y"=0.0} ("Rotation Center From Robot Center") T33 {"X"=28.0, "Y"=0.0} ("Rotation Center From Robot Center")] -> w165
    frame False {
      # "Rotation center at center"
    }
    frame True {
      # "Move out rotation center"
    }
  }
  n170 = global read "Global_ACT_Data Out.vi" "ACT_Wrist_HW Output"() -> (→"ACT_Wrist_HW Output":T5)
  n171 = global read "Global_ACT_Data Out.vi" "ACT_Extend_HW Outputs"() -> (→"ACT_Extend_HW Outputs":T12)
  n172 = global read "Global_ACT_Data Out.vi" "ACT_Lift_HW Outputs"() -> (→"ACT_Lift_HW Outputs":T11)
  n173 = Bundle By Name(cluster=T31 {"Mode"=enum."Coast", "Direction"={"Traverse"={"Velocity"=0.0, "Angle"=0.0, "Rotations Count"=0.0}, "Rotate(Yaw) CCW 1 CW -1"=0.0}, "Orientation Robot(t) Field(f)"=FALSE, "Max Translation Speed (ft/sec)"=0.0, "Rotation Reduction 1-0"=0.0, "Rotation Center From Robot Center"={"X"=0.0, "Y"=0.0}, "Auto Angle"=0.0, "Auto Target (ft)"=0.0} ("CMD_ACT_Template_Data"), "Rotation Center From Robot Center"=w165, "Max Translation Speed (ft/sec)"=w7, "Orientation Robot(t) Field(f)"=FALSE, "Mode"=w6, "Rotation Reduction 1-0"=w9, "Direction.Rotate(Yaw) CCW 1 CW -1"=w82, "Direction.Traverse"=w8, "Auto Angle"=w3, "Auto Target (ft)"=w10) -> (w177:T31)
  n174 = Index Array(array=w142, index=w172) -> (element=w173:bool)
  n175 = Bundle By Name(cluster=T28 {"Reset"=FALSE, "Disable"=FALSE} ("CMD_SEN_Pigeon_Data"), "Reset"=w173, "Disable"=FALSE) -> (w174:T28)
  n176 = global write "Global_CMD_ACT_Data In.vi" "CMD_ACT_SwerveDrive_Data"(w177) -> ()
  n177 = global write "Global_CMD_SEN_Data In.vi" "CMD_SEN_Pigeon_Data"(w174) -> ()
  n178 = global write "Global_CMD_Data In.vi" "CMD_SEN_GameController_BUZZ Select"(w37) -> ()
  n179 = global write "Global_CMD_Data In.vi" "CMD_SEN_GameController_BUZZNumber"(w36) -> ()
  n180 = call-poly <vilib>:"NT Write Value.vi"("name"="RobotDrive Motors" ("Name")) -> ()  [unwired: 10 in, 1 out]
  n181 = call-poly <vilib>:"NT Write Value.vi"("name"="Joystick 0/Axes" ("Name")) -> ()  [unwired: 10 in, 1 out]
  n182 = call-poly <vilib>:"NT Write Value.vi"("name"="Joystick 0/Buttons" ("Name")) -> ()  [unwired: 10 in, 1 out]
